vi "Update.vi"(8 "error in (no error)":errorcluster, 10 "Message in":refnum<class "UpdateMessage.lvclass">, 11 "TomoConversion in":refnum<class "TomoConversion.lvclass">) -> (0 "error out":errorcluster, 3 "TomoConversion out":refnum<class "TomoConversion.lvclass">)   [LabVIEW 2012, in "TomoConversion.lvclass"]
doc: "The update method processes the command 'update'. \n\nThe command 'update' is used for receiving new values to be set to the private data of the class. This could be seen as a public set method for setting new parameters to the private class data."
uses:
  TomoConversion.lvclass
  <vilib>/Distrio/Murmex/UpdateMessage/UpdateMessage.lvclass
  TomoConversion.lvclass/TomoConversion.ctl
  <vilib>/Distrio/Murmex/Murmex/Murmex.lvclass
panel:
  # "This method is called when the UPDATE\ntrigger is sent. \n\nOverride this method when your component needs to\nrespond to this trigger. \n\nCall parent for proper implementation"
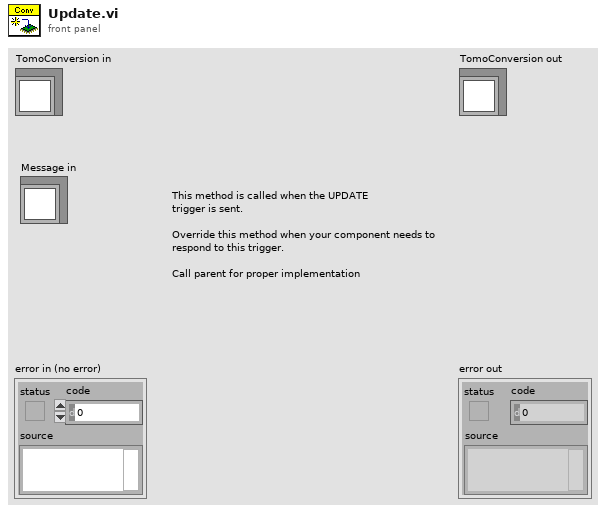
[diagram p1: front panel]
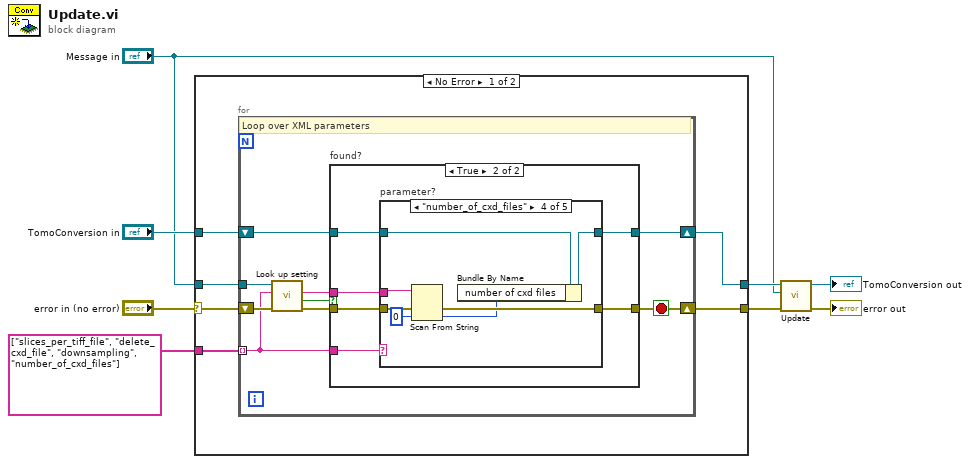
[diagram p0: block diagram]
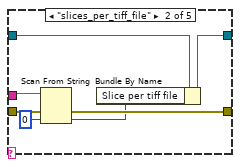
[diagram p4: hidden frame]
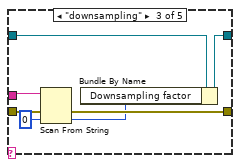
[diagram p5: hidden frame]
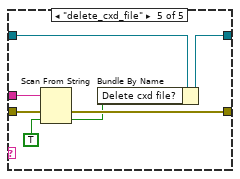
[diagram p6: hidden frame]
diagram:
  n1 = case shown="No Error" "error in (no error)" {
    selector: "error in (no error)" -> [w14 w62]
    tunnel: "Message in" -> [w13 _]
    tunnel: string[] ["slices_per_tiff_file", "delete_cxd_file", "downsampling", "number_of_cxd_files"] -> [w12 _]
    tunnel: "TomoConversion in" -> [w11 w63]
    tunnel: [w10 w62] -> w4
    tunnel: [w9 w63] -> w3
    frame No Error {
      n2 = for {
        tunnel: w13 -> [w22]
        tunnel: w12 -> [w15] mode=indexing
        shift-right: [w19] -> w10
        shift-left: w14 -> [w23]
        shift-right: [w18] -> w9
        shift-left: w11 -> [w17]
        stop <- w19 stop-if-true
        # "Loop over XML parameters"
        n3 = call <vilib>:"Look up setting.vi"("error in (no error)"=w23, "tag name"=w15, "UpdateMessage in"=w22) -> ("error out"=w20:errorcluster, "found?"=w21:bool, "value"=w16:string)  [unwired: 5 in, 1 out]
        n4 = case "found?" shown="True" w21 {
          tunnel: w20 -> [w25 w28]
          tunnel: [w25 w29] -> w19
          tunnel: [w24 w31] -> w18
          tunnel: w17 -> [w24 w30]
          tunnel: w16 -> [_ w26]
          tunnel: w15 -> [_ w27]
          frame False {
          }
          frame True {
            n5 = case "parameter?" shown="\"number_of_cxd_files\"" w27 {
              tunnel: [w33 w39 w46 w53 w60] -> w31
              tunnel: w30 -> [w33 w40 w47 w54 w61]
              tunnel: [w32 w37 w44 w51 w58] -> w29
              tunnel: w28 -> [w32 w38 w45 w52 w59]
              tunnel: w26 -> [_ w35 w42 w49 w57]
              frame Default {
              }
              frame "slices_per_tiff_file" {
                n6 = Scan From String(input string=w35, error in=w38, default 1=u32 0 ("default value 1")) -> (error out=w37:errorcluster, output 1=w36:u32)  [unwired: 2 in, 2 out]
                n7 = Bundle By Name(cluster=w40, "Slice per tiff file"=w36) -> (w39:refnum<class "TomoConversion.lvclass">)
              }
              frame "downsampling" {
                n8 = Scan From String(input string=w42, error in=w45, default 1=u32 0 ("default value 1")) -> (error out=w44:errorcluster, output 1=w43:u32)  [unwired: 2 in, 2 out]
                n9 = Bundle By Name(cluster=w47, "Downsampling factor"=w43) -> (w46:refnum<class "TomoConversion.lvclass">)
              }
              frame "number_of_cxd_files" {
                n10 = Scan From String(input string=w49, error in=w52, default 1=0 ("default value 1")) -> (error out=w51:errorcluster, output 1=w50:i32)  [unwired: 2 in, 2 out]
                n11 = Bundle By Name(cluster=w54, "number of cxd files"=w50) -> (w53:refnum<class "TomoConversion.lvclass">)
              }
              frame "delete_cxd_file" {
                n12 = Scan From String(input string=w57, error in=w59, default 1=TRUE) -> (error out=w58:errorcluster, output 1=w56:bool)  [unwired: 2 in, 2 out]
                n13 = Bundle By Name(cluster=w61, "Delete cxd file?"=w56) -> (w60:refnum<class "TomoConversion.lvclass">)
              }
            }
          }
        }
      }
    }
    frame Error {
    }
  }
  n14 = call-parent "Update.vi"("error in (no error)"=w4, "Message in"="Message in", "Murmex in"=w3) -> ("error out"=→"error out":errorcluster, "Murmex out"=→"TomoConversion out":refnum<class "TomoConversion.lvclass">)  [unwired: 7 in]
